vi "Test Configure.vi"(0 "Template Tx Test in":refnum<class "niDTS Calibration Cal IsNeeded RF Test.lvclass">, 11 "error in (no error)":errorcluster) -> (4 "Template Tx Test out":refnum<class "niDTS Calibration Cal IsNeeded RF Test.lvclass">, 15 "error out":errorcluster)   [LabVIEW 2015, in "niDTS Utilities.lvlib" / "niDTS Calibration Cal IsNeeded RF Test.lvclass"]
uses:
  niDTS Calibration Cal IsNeeded RF Test.lvclass
  niDTS Calibration Cal IsNeeded RF Test.lvclass/niDTS Calibration Cal IsNeeded RF Test.ctl
  Properties/Calibration Cal IsNeeded Set Ports.vi
  Properties/Calibration Cal IsNeeded Set InstDriver Handle in.vi
  TestStand/Station/Objects/SystemTechnologyCatalog/niDTS SystemTechnologyCatalog.lvclass
  TestStand/Station/Objects/SystemDut/niDTS SystemDut.lvclass
  RiviInstDriver/niRfGeneralSettings/Objects/niRfGeneralSettings.lvclass
  TestStand/niDTS TestStand.lvlib
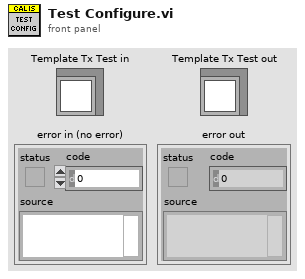
[diagram p1: front panel]
types:
  T1 = typedef "niDTS Utilities.lvlib/niDTS Calibration Cal IsNeeded RF Test INC Parameters.ctl" = cluster{"Temperature Change":dbl, "Time Range":i32}
  T2 = typedef "InstDriver.lvclass/niInstDriver INC Handle.ctl" = refnum<data-value>
  T3 = typedef "niRfGeneralSettings.lvclass/niRfGeneralSettings INC Handle.ctl" = refnum<data-value>
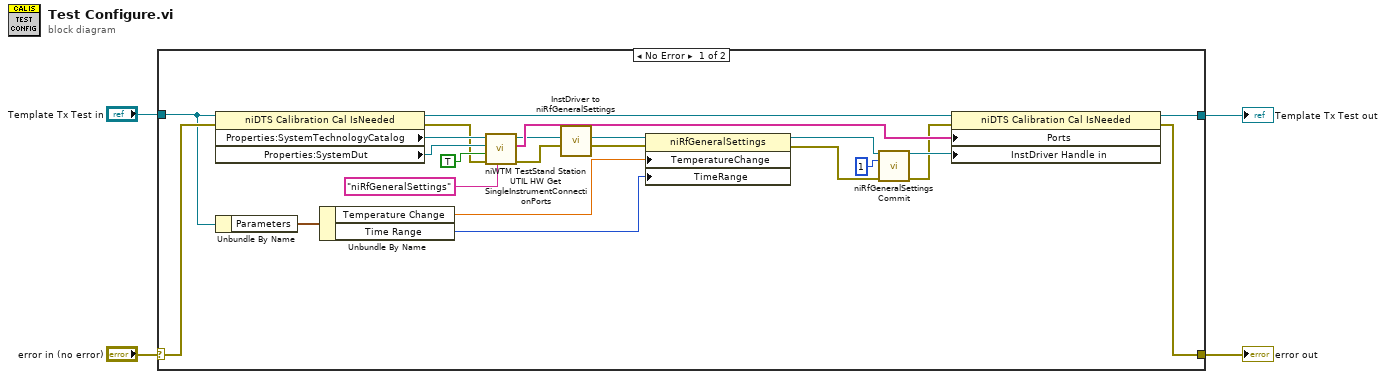
[diagram p0: block diagram]
diagram:
  n1 = case shown="No Error" "error in (no error)" {
    selector: "error in (no error)" -> [w23 w29]
    tunnel: [w22 w29] -> w3
    tunnel: "Template Tx Test in" -> [w15 w28]
    tunnel: [w21 w28] -> w1
    frame No Error {
      n2 = property class="niDTS Calibration Cal IsNeeded "(reference=w15, error in=w23) -> (reference out=w14:refnum<class "niDTS Calibration Cal IsNeeded RF Test.lvclass">, error out=w24:errorcluster, "Properties:SystemTechnologyCatalog"=w27:refnum<class "niDTS SystemTechnologyCatalog.lvclass">, "Properties:SystemDut"=w26:refnum<class "niDTS SystemDut.lvclass">)
      n3 = Unbundle By Name(w15) -> ("Parameters"=w20:T1)
      n4 = Unbundle By Name(w20) -> ("Temperature Change"=w10:dbl, "Time Range"=w9:i32)
      n5 = call "niWTM TestStand Station UTIL HW Get SingleInstrumentConnectionPorts.vi"("InstDriver Name"="niRfGeneralSettings", "error in (no error)"=w24, "TX Instrument"=TRUE, "SystemDut"=w26, "SystemTechnologyCatalog"=w27) -> ("error out"=w12:errorcluster, "Ports"=w17:string[], "InstDriver Handle"=w13:T2)  [unwired: 4 in]
      n6 = call "InstDriver to niRfGeneralSettings.vi"("error in (no error)"=w12, "InstDriver Handle in"=w13) -> ("error out"=w6:errorcluster, "InstDriver Handle out"=w11:refnum<data-value>)  [unwired: 8 in]
      n7 = property class="niRfGeneralSettings"(reference=w11, error in=w6, "TemperatureChange"=w10, "TimeRange"=w9) -> (reference out=w8:refnum<data-value>, error out=w7:errorcluster)
      n8 = call "niRfGeneralSettings Commit.vi"("InstDriver Handle in"=w8, "Instance"=1, "error in (no error)"=w7) -> ("InstDriver Handle out"=w18:T3, "error out"=w16:errorcluster)  [unwired: 11 in]
      n9 = property class="niDTS Calibration Cal IsNeeded "(reference=w14, error in=w16, "Ports"=w17, "InstDriver Handle in"=w18) -> (reference out=w21:refnum<class "niDTS Calibration Cal IsNeeded RF Test.lvclass">, error out=w22:errorcluster)
    }
    frame Error {
    }
  }
  "error out" <- w3
  "Template Tx Test out" <- w1
